vi "Init_Dot_Matrix_With_Statuses-1.vi"(1 "[IN] Initial (X,Y) matrix":dbl[][](array[numeric])) -> (0 "[OUT] Dot matrix\nwith initial status":i16[][](array[numeric]))   [LabVIEW 2013]
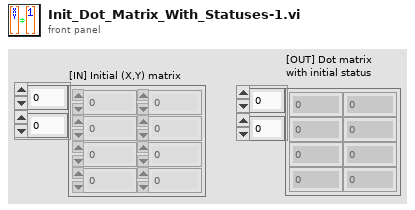
[diagram p1: front panel]
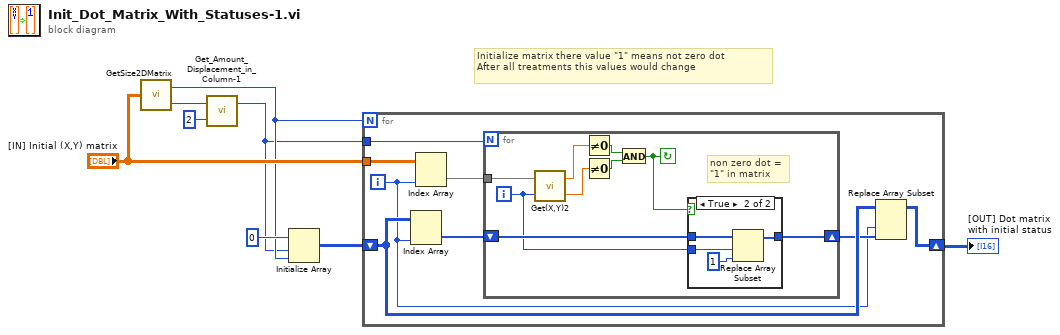
[diagram p0: block diagram]
diagram:
  # "Initialize matrix there value \"1\" means not zero dot\nAfter all treatments this values would change"
  n1 = call "GetSize2DMatrix.vi"("Array IN (2D)"="[IN] Initial (X,Y) matrix") -> ("# Cols"=w2:i32, "# Rows"=w3:i32)
  n2 = call "Get_Amount_Displacement_in_Column-1.vi"("multiplier"=2 ("y"), "# Rows"=w3) -> ("Displ amount"=w1:i32)  [unwired: 1 out]
  n3 = Initialize Array(i16 0 ("element"), w1, w2) -> (w7:i16[][])
  n4 = for {
    N: w2 -> [_]
    shift-right: [w10] -> w5
    shift-left: w7 -> [w12]
    tunnel: "[IN] Initial (X,Y) matrix" -> [w16]
    tunnel: w1 -> [w15]
    i -> [w9]
    n5 = Index Array(array=w12, index (col)=w9) -> (element=w13:i16[])  [unwired: 1 in]
    n6 = Index Array(array=w16, index (col)=w9) -> (element=w14:dbl[])  [unwired: 1 in]
    n7 = for {
      N: w15 -> [_]
      tunnel: w14 -> [w20]
      shift-right: [w21] -> w11
      shift-left: w13 -> [w22]
      i -> [w19]
      stop <- w23 continue-if-true
      # "non zero dot =\n\"1\" in matrix"
      n8 = call "Get(X,Y)2.vi"("[IN] index of (X,Y)"=w19, "[IN] Array coordi\nnates (X,Y) in Frame"=w20) -> ("[OUT] Y"=w17:dbl, "[OUT] X"=w18:dbl)
      n9 = Not Equal To 0?(x=w18) -> (x != 0?=w25:bool)
      n10 = Not Equal To 0?(x=w17) -> (x != 0?=w24:bool)
      n11 = And(x=w25, y=w24) -> (x .and. y?=w23:bool)
      n12 = case shown="True" w23 {
        tunnel: w22 -> [w26 w30]
        tunnel: w19 -> [_ w29]
        tunnel: [w26 w27] -> w21
        frame False {
        }
        frame True {
          n13 = Replace Array Subset(array=w30, new element=i16 1 ("new element/subarray"), index=w29) -> (w27:i16[])
        }
      }
    }
    n14 = Replace Array Subset(array=w12, new element=w11, index (col)=w9) -> (w10:i16[][])  [unwired: 1 in]
  }
  "[OUT] Dot matrix\nwith initial status" <- w5
